vi "putNodeInOpen.vi"(8 "error in (no error)":errorcluster, 9 "SearchMethod":T1, 10 "GraphNode":refnum<data-value>, 11 "Graph in":refnum<class "Graph.lvclass">) -> (0 "error out":errorcluster, 3 "Graph out":refnum<class "Graph.lvclass">)   [LabVIEW 2014, in "Graph.lvlib" / "Graph.lvclass"]
doc: "Puts a node in the sorted list OPEN. OPEN keeps track which nodes are left to search through. The front of the list OPEN are the nodes we are planning on searching the soonest. After you expand the search, the nodes are placed in OPEN. Each method defines a different way of putting nodes in the OPEN.s"
uses:
  <userlib>/AdvancedDataStructures/ClassBased/Graph/Graph.lvclass
  <userlib>/AdvancedDataStructures/ClassBased/Graph/SearchMethod.ctl
  <userlib>/AdvancedDataStructures/ClassBased/GraphNode/GraphNode.lvclass
  <userlib>/AdvancedDataStructures/ClassBased/Graph/Graph.lvclass/Graph.ctl
  <userlib>/AdvancedDataStructures/ClassBased/LinkedList/position.ctl
  <userlib>/AdvancedDataStructures/ClassBased/LinkedList/InsertSearchOptions.ctl
  <userlib>/AdvancedDataStructures/ClassBased/LinkedList/LinkedList.lvclass
  <userlib>/AdvancedDataStructures/ClassBased/Common/BasicSortedList/BasicSortedList/BasicSortedList.lvclass
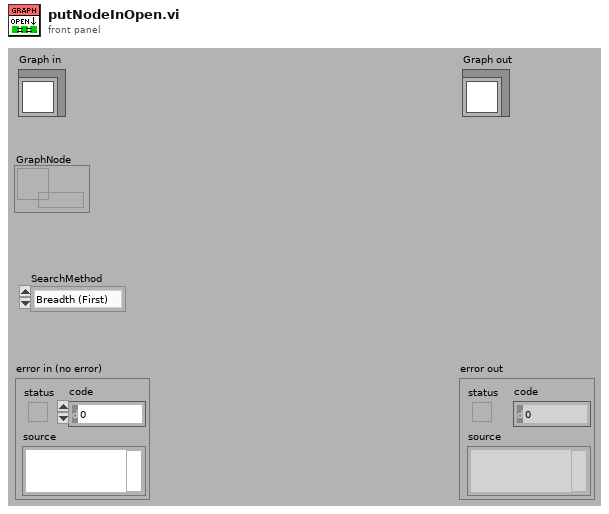
[diagram p1: front panel]
types:
  T1 = typedef "Graph.lvlib/Graph.lvclass/SearchMethod.ctl" = enum16{"Breadth (First)", "Depth (First)", "Best First", "Breadth (Best)", "Depth (Best)"}
  T2 = typedef "LinkedList.lvlib/LinkedList.lvclass/position.ctl" = enum16{"Front", "Back", "Search"}
  T3 = typedef "LinkedList.lvlib/LinkedList.lvclass/InsertSearchOptions.ctl" = cluster{"InsertIfEmpty":bool, "Insert After":bool, "InsertIfNotFound":bool}
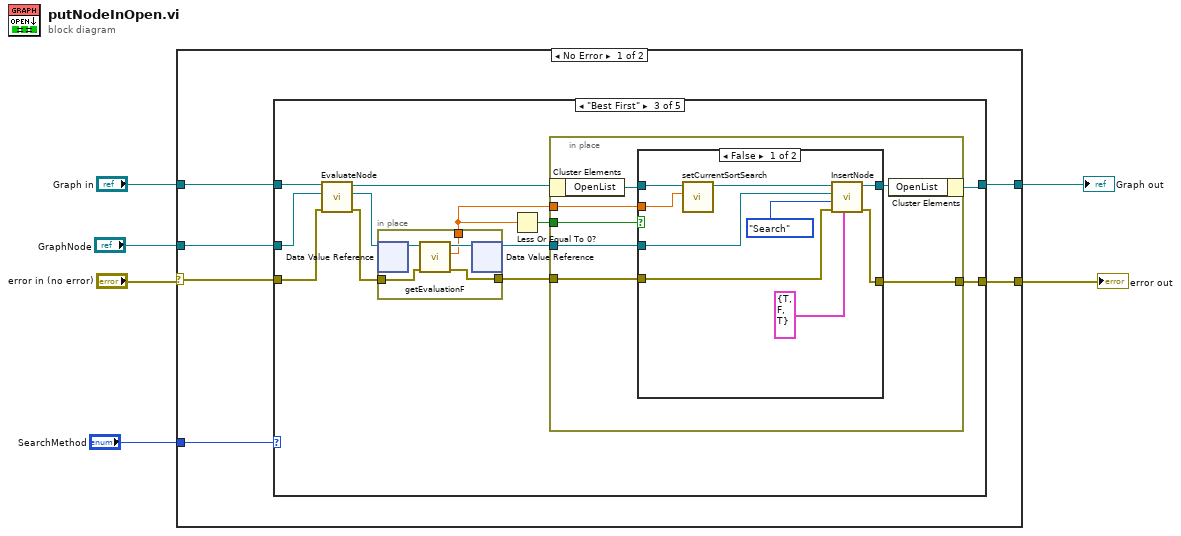
[diagram p0: block diagram]
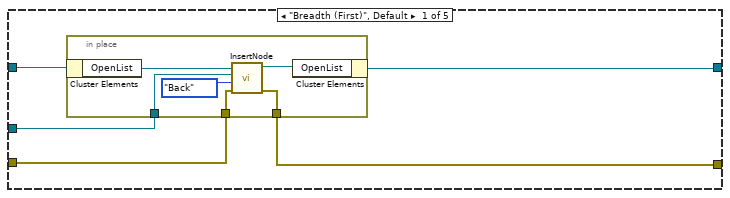
[diagram p2: hidden frame]
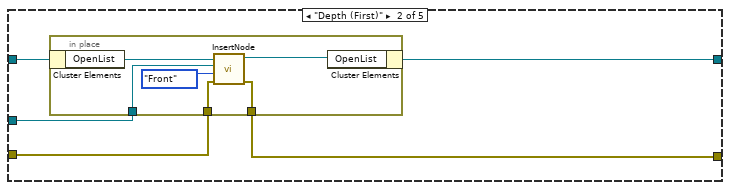
[diagram p3: hidden frame]
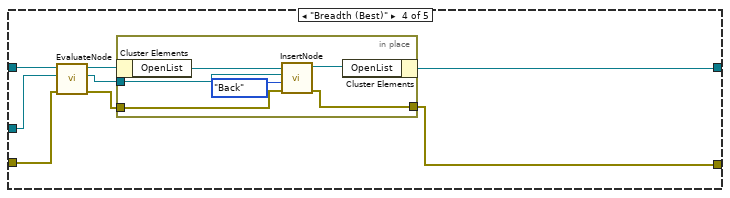
[diagram p5: hidden frame]
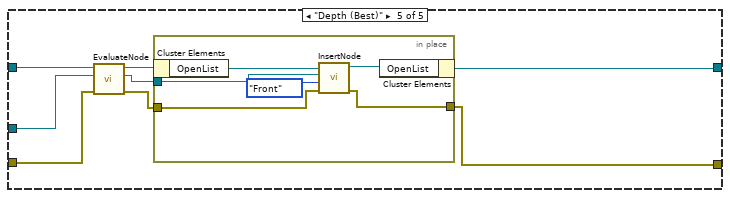
[diagram p6: hidden frame]
diagram:
  n1 = case shown="No Error" "error in (no error)" {
    selector: "error in (no error)" -> [w8 w99]
    tunnel: [w11 w99] -> w1
    tunnel: [w7 w98] -> w2
    tunnel: "Graph in" -> [w10 w98]
    tunnel: "GraphNode" -> [w9 _]
    tunnel: "SearchMethod" -> [w12 _]
    frame No Error {
      n2 = case shown="\"Best First\"" w12 {
        tunnel: w9 -> [w17 w28 w40 w75 w85]
        tunnel: w8 -> [w16 w27 w39 w76 w86]
        tunnel: [w15 w26 w45 w70 w84] -> w11
        tunnel: w10 -> [w14 w25 w41 w77 w88]
        tunnel: [w13 w24 w35 w73 w87] -> w7
        frame "Breadth (First)", Default {
          n3 = in-place {
            in-place-border: w17 -> [w23]
            in-place-border: w16 -> [w22]
            in-place-border: [w20] -> w15
            n4 = in-place-cluster #1(w14) -> ("OpenList"=w19:refnum<class "BasicSortedList.lvclass">)
            n5 = call <userlib>:"InsertNode.vi"("error in (no error)"=w22, "position"=position."Back", "ToInsert"=w23, "LinkedList in"=w19) -> ("error out"=w20:errorcluster, "LinkedList out"=w18:refnum<class "BasicSortedList.lvclass">)  [unwired: 5 in, 1 out]
            n6 = in-place-cluster #1("OpenList"=w18) -> (w13:refnum<class "Graph.lvclass">)
          }
        }
        frame "Depth (First)" {
          n7 = in-place {
            in-place-border: w28 -> [w33]
            in-place-border: w27 -> [w32]
            in-place-border: [w31] -> w26
            n8 = in-place-cluster #2(w25) -> ("OpenList"=w30:refnum<class "BasicSortedList.lvclass">)
            n9 = call <userlib>:"InsertNode.vi"("error in (no error)"=w32, "position"=position."Front", "ToInsert"=w33, "LinkedList in"=w30) -> ("error out"=w31:errorcluster, "LinkedList out"=w29:refnum<class "BasicSortedList.lvclass">)  [unwired: 5 in, 1 out]
            n10 = in-place-cluster #2("OpenList"=w29) -> (w24:refnum<class "Graph.lvclass">)
          }
        }
        frame "Best First" {
          n11 = call <userlib>:"EvaluateNode.vi"("error in (no error)"=w39, "ToEvaluate in"=w40, "Graph in"=w41) -> ("error out"=w37:errorcluster, "ToEvaluate out"=w38:refnum<data-value>, "Graph out"=w36:refnum<class "Graph.lvclass">)  [unwired: 6 in]
          n12 = in-place {
            in-place-border: [w68] -> w43
            in-place-border: [w67] -> w46
            in-place-border: w37 -> [w66]
            n13 = in-place-dvr #3(w38) -> (w65:refnum<class "GraphNode.lvclass">)  [unwired: 1 out]
            n14 = call <userlib>:"getEvaluationF.vi"("error in (no error)"=w66, "GraphNode in"=w65) -> ("error out"=w67:errorcluster, "F"=w68:dbl, "GraphNode out"=w69:refnum<class "GraphNode.lvclass">)  [unwired: 7 in]
            n15 = in-place-dvr #3(w69) -> (w44:refnum<data-value>)  [unwired: 1 out]
          }
          n16 = Less Or Equal To 0?(x=w43) -> (x <= 0?=w42:bool)
          n17 = in-place {
            in-place-border: w46 -> [w53]
            in-place-border: [w52] -> w45
            in-place-border: w44 -> [w51]
            in-place-border: w43 -> [w50]
            in-place-border: w42 -> [w49]
            n18 = in-place-cluster #4(w36) -> ("OpenList"=w48:refnum<class "BasicSortedList.lvclass">)
            n19 = case shown="False" w49 {
              tunnel: w48 -> [w56 w64]
              tunnel: [w62 w64] -> w47
              tunnel: w53 -> [w57 w63]
              tunnel: [w60 w63] -> w52
              tunnel: w51 -> [w59 _]
              tunnel: w50 -> [w54 _]
              frame False {
                n20 = call <userlib>:"setCurrentSortSearch.vi"("CurrentSortSearch"=w54, "BasicSortedList in"=w56) -> ("BasicSortedList out"=w55:refnum<class "BasicSortedList.lvclass">)  [unwired: 8 in, 1 out]
                n21 = call <userlib>:"InsertNode.vi"("Insert Search"=T3 {"InsertIfEmpty"=TRUE, "Insert After"=FALSE, "InsertIfNotFound"=TRUE}, "error in (no error)"=w57, "position"=position."Search", "ToInsert"=w59, "LinkedList in"=w55) -> ("error out"=w60:errorcluster, "LinkedList out"=w62:refnum<class "BasicSortedList.lvclass">)  [unwired: 4 in, 1 out]
              }
              frame True {
              }
            }
            n22 = in-place-cluster #4("OpenList"=w47) -> (w35:refnum<class "Graph.lvclass">)
          }
        }
        frame "Breadth (Best)" {
          n23 = call <userlib>:"EvaluateNode.vi"("error in (no error)"=w76, "ToEvaluate in"=w75, "Graph in"=w77) -> ("error out"=w71:errorcluster, "ToEvaluate out"=w72:refnum<data-value>, "Graph out"=w74:refnum<class "Graph.lvclass">)  [unwired: 6 in]
          n24 = in-place {
            in-place-border: w72 -> [w83]
            in-place-border: w71 -> [w78]
            in-place-border: [w81] -> w70
            n25 = in-place-cluster #5(w74) -> ("OpenList"=w80:refnum<class "BasicSortedList.lvclass">)
            n26 = call <userlib>:"InsertNode.vi"("error in (no error)"=w78, "position"=position."Back", "ToInsert"=w83, "LinkedList in"=w80) -> ("error out"=w81:errorcluster, "LinkedList out"=w79:refnum<class "BasicSortedList.lvclass">)  [unwired: 5 in, 1 out]
            n27 = in-place-cluster #5("OpenList"=w79) -> (w73:refnum<class "Graph.lvclass">)
          }
        }
        frame "Depth (Best)" {
          n28 = call <userlib>:"EvaluateNode.vi"("error in (no error)"=w86, "ToEvaluate in"=w85, "Graph in"=w88) -> ("error out"=w89:errorcluster, "ToEvaluate out"=w90:refnum<data-value>, "Graph out"=w91:refnum<class "Graph.lvclass">)  [unwired: 6 in]
          n29 = in-place {
            in-place-border: w90 -> [w97]
            in-place-border: w89 -> [w92]
            in-place-border: [w95] -> w84
            n30 = in-place-cluster #6(w91) -> ("OpenList"=w94:refnum<class "BasicSortedList.lvclass">)
            n31 = call <userlib>:"InsertNode.vi"("error in (no error)"=w92, "position"=position."Front", "ToInsert"=w97, "LinkedList in"=w94) -> ("error out"=w95:errorcluster, "LinkedList out"=w93:refnum<class "BasicSortedList.lvclass">)  [unwired: 5 in, 1 out]
            n32 = in-place-cluster #6("OpenList"=w93) -> (w87:refnum<class "Graph.lvclass">)
          }
        }
      }
    }
    frame Error {
    }
  }
  "error out" <- w1
  "Graph out" <- w2
